vi "Practica 01.vi"() -> ()   [LabVIEW 2011]
panel:
  out "Alarma":bool
  in  "PUERTO SERIAL":refnum<visa-resource-name>
  in  "stop":bool
  in  "Frecuencia":u32(knob) caption="Frecuencia del tren de pulsos (kHz)" scale=0.0..150.0
  in  "Dirección":bool
  in  "SERVO ON":bool
  # "Deslizador Lineal UTN"
  # "CONTOL DE POSICIÓN"
  # "PRUEBAS BÁSICAS CON EL SERVOMOTOR"
  # "kHz"
  # "PTO:"
  # "1. Encender el servomotor"
  # "2. Especificar la frecuenca del \n    tren de pulsos"
  # "3. Cambio de dirección de giro"
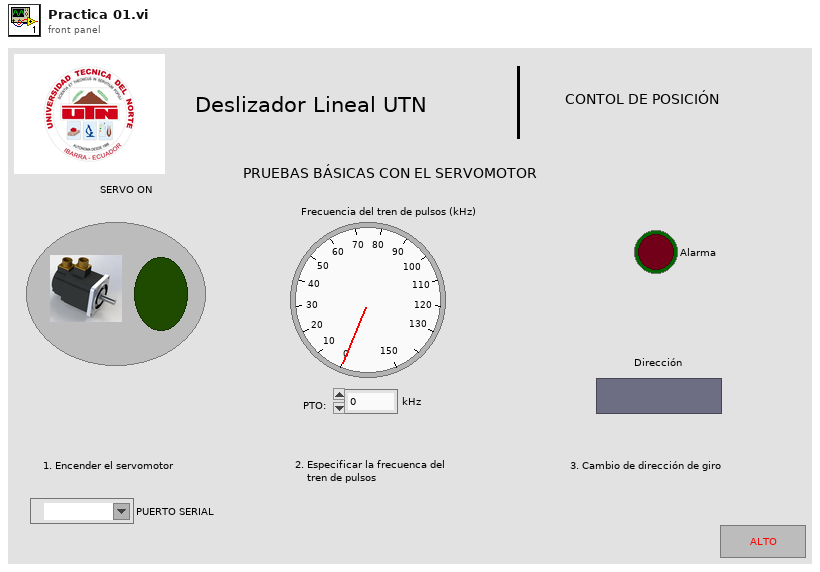
[diagram p1: front panel]
types:
  T1 = enum16{"Aout", "Fout", "Direccion", "ServoOn", "Idle"}
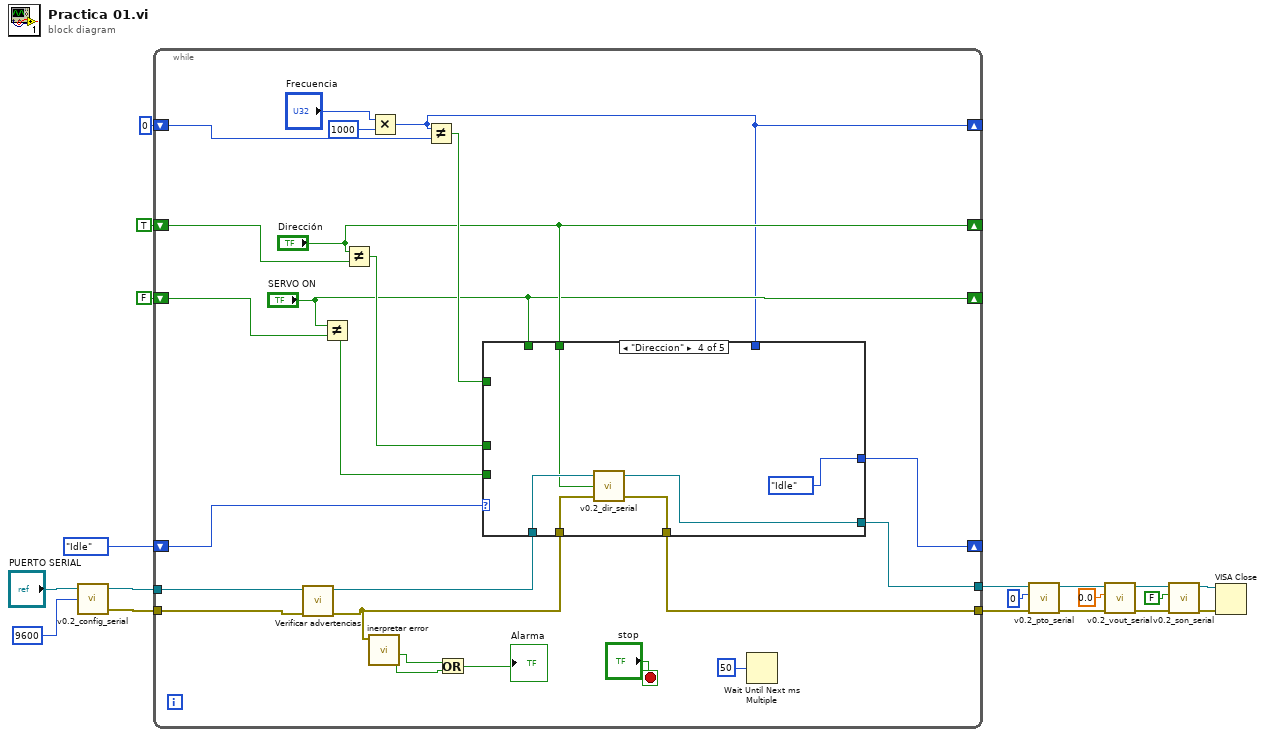
[diagram p0: block diagram]
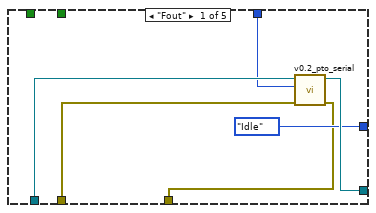
[diagram p2: hidden frame]
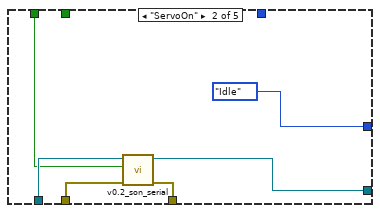
[diagram p3: hidden frame]
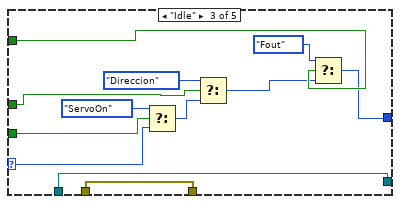
[diagram p4: hidden frame]
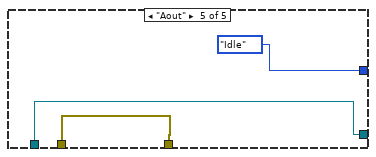
[diagram p5: hidden frame]
diagram:
  n1 = call "v0.2_config_serial.vi"("baud rate (9600/115200)"=u32 9600, "VISA COM IN"="PUERTO SERIAL") -> ("error out"=w17:errorcluster, "VISA COM OUT"=w18:refnum<visa-resource-name>)  [unwired: 2 in]
  n2 = while {
    tunnel: w18 -> [w26]
    tunnel: w17 -> [w25]
    shift-right: [w27] -> _
    shift-left: u32 0 ("Fout") -> [w42]
    tunnel: [w30] -> w8
    shift-right: [w38] -> _
    shift-left: T1."Idle" -> [w40]
    shift-right: ["Dirección"] -> _
    shift-left: TRUE ("Direccion") -> [w37]
    shift-right: ["SERVO ON"] -> _
    shift-left: FALSE ("SON") -> [w35]
    tunnel: [w33] -> w12
    stop <- "stop" stop-if-true
    n3 = call "Verificar advertencias.vi"("error in"=w25, "VISA COM IN"=w26) -> ("error out"=w23:errorcluster, "VISA COM OUT"=w24:refnum<visa-resource-name>)  [unwired: 8 in]
    n4 = Not Equal?(x="SERVO ON", y=w35) -> (x != y?=w34:bool)
    n5 = Not Equal?(x="Dirección", y=w37) -> (x != y?=w36:bool)
    n6 = call "inerpretar error.vi"("error out"=w23) -> ("Alarma Proximidad Encoder"=w21:bool, "Alarma Proximidad MOtor"=w22:bool)  [unwired: 5 in, 4 out]
    n7 = Multiply(x="Frecuencia", y=u32 1000) -> (x*y=w27:u32)
    n8 = Not Equal?(x=w27, y=w42) -> (x != y?=w39:bool)
    n9 = Or(x=w22, y=w21) -> (x .or. y?=→"Alarma":bool)
    n10 = case shown="\"Direccion\"" w40 {
      selector: w40 -> [_ _ w61 _ _]
      tunnel: w39 -> [_ _ w67 _ _]
      tunnel: [T1."Idle" T1."Idle" w65 T1."Idle" T1."Idle"] -> w38
      tunnel: w36 -> [_ _ w59 _ _]
      tunnel: w34 -> [_ _ w60 _ _]
      tunnel: w24 -> [w49 w55 w58 w73 w75]
      tunnel: w27 -> [w48 _ _ _ _]
      tunnel: [w47 w53 w58 w71 w75] -> w33
      tunnel: "SERVO ON" -> [_ w54 _ _ _]
      tunnel: "Dirección" -> [_ _ _ w72 _]
      tunnel: w23 -> [w45 w51 w57 w69 w76]
      tunnel: [w44 w50 w57 w68 w76] -> w30
      frame "Fout" {
        n11 = call "v0.2_pto_serial.vi"("error in (no error)"=w45, "Fout"=w48, "VISA COM IN"=w49) -> ("error out"=w44:errorcluster, "VISA COM OUT"=w47:refnum<visa-resource-name>)  [unwired: 7 in]
      }
      frame "ServoOn" {
        n12 = call "v0.2_son_serial.vi"("error in (no error)"=w51, "ServoON"=w54, "VISA COM IN"=w55) -> ("error out"=w50:errorcluster, "VISA COM OUT"=w53:refnum<visa-resource-name>)  [unwired: 7 in]
      }
      frame "Idle" {
        n13 = Select(t=T1."ServoOn", s=w60, f=w61) -> (s? t:f=w62:T1)
        n14 = Select(t=T1."Direccion", s=w59, f=w62) -> (s? t:f=w56:T1)
        n15 = Select(t=T1."Fout", s=w67, f=w56) -> (s? t:f=w65:T1)
      }
      frame "Direccion" {
        n16 = call "v0.2_dir_serial.vi"("error in (no error)"=w69, "Direccion"=w72, "VISA COM IN"=w73) -> ("error out"=w68:errorcluster, "VISA COM OUT"=w71:refnum<visa-resource-name>)  [unwired: 1 in]
      }
      frame "Aout" {
      }
    }
    n17 = Wait Until Next ms Multiple(millisecond multiple=u32 50) -> ()  [unwired: 1 out]
  }
  n18 = call "v0.2_pto_serial.vi"("error in (no error)"=w8, "Fout"=u32 0, "VISA COM IN"=w12) -> ("error out"=w7:errorcluster, "VISA COM OUT"=w11:refnum<visa-resource-name>)  [unwired: 7 in]
  n19 = call "v0.2_vout_serial.vi"("error in (no error)"=w7, "Volt"=0.0, "VISA COM IN"=w11) -> ("error out"=w6:errorcluster, "VISA COM OUT"=w10:refnum<visa-resource-name>)  [unwired: 7 in]
  n20 = call "v0.2_son_serial.vi"("error in (no error)"=w6, "ServoON"=FALSE, "VISA COM IN"=w10) -> ("error out"=w5:errorcluster, "VISA COM OUT"=w9:refnum<visa-resource-name>)  [unwired: 7 in]
  n21 = VISA Close(VISA resource name=w9, error in (no error)=w5) -> ()  [unwired: 1 out]
